vi "abort.vi"(8 "error in (no error)":errorcluster caption="错误输入（无错误）", 11 "虚拟 输入":refnum<class "虚拟.lvclass">) -> (0 "error out":errorcluster caption="错误输出", 3 "虚拟 输出":refnum<class "虚拟.lvclass">)   [LabVIEW 2020, in "虚拟.lvclass"]
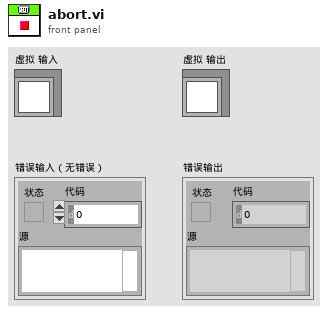
[diagram p1: front panel]
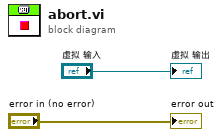
[diagram p0: block diagram]
diagram:
  "error out" <- "error in (no error)"
  "虚拟 输出" <- "虚拟 输入"
